vi "sub_associate_token.vi"(8 "error in":errorcluster, 9 "save to device?":bool=TRUE, 10 "device_id":string, 11 "daq.io type in":T1) -> (0 "error out":errorcluster, 3 "daq.io type out":T1={"daq.io ref"=refnum, "daq.io API Base"="http://dashboard.daq.io/api/v1", "Device Key"="", "Account ID"="", "online"=TRUE, "SSL"=TRUE})   [LabVIEW 2013, in "daqio minimal.lvlib"]
doc: "This VI associates the current token with the specified device. If \"save to device\" is true, it will also register the token on the device (default behavior)"
uses:
  daqio minimal.lvlib
  _typedefs/daqio-Type.ctl
  <vilib>/httpClient/ClientHandle.ctl
  <vilib>/Easy HTTP Client/Easy HTTP.lvlib
  <vilib>/httpClient/LabVIEWHTTPClient.lvlib
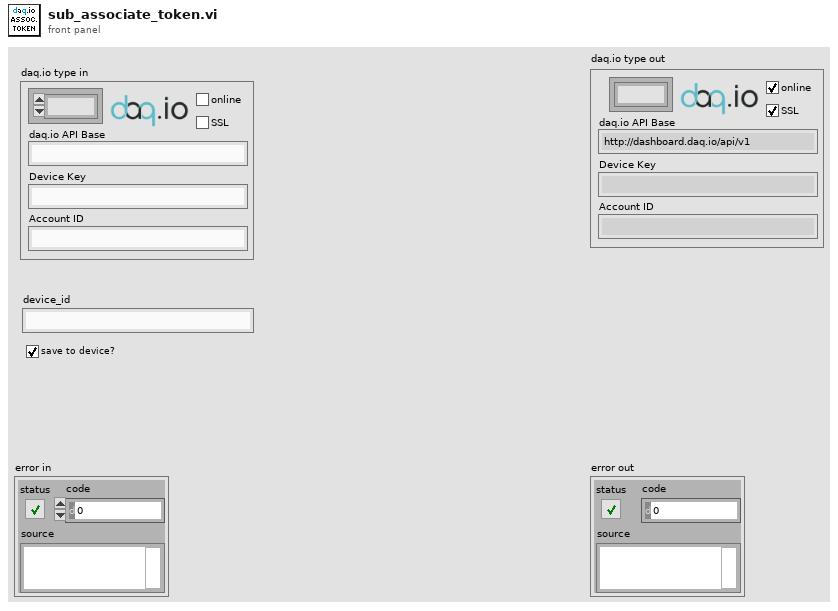
[diagram p1: front panel]
types:
  T1 = typedef "daqio minimal.lvlib/daqio-Type.ctl" = cluster{"daq.io ref":T2, "daq.io API Base":string, "Device Key":string, "Account ID":string, "online":bool, "SSL":bool}
  T2 = typedef "LabVIEWHTTPClient.lvlib/ClientHandle.ctl" = refnum<k1>
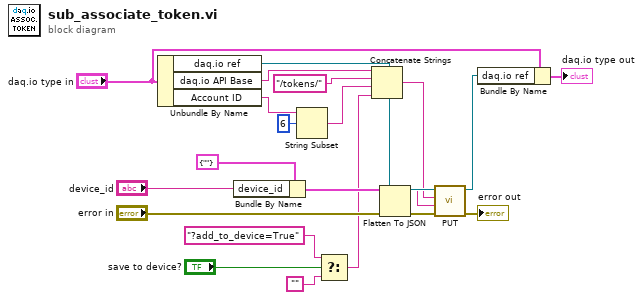
[diagram p0: block diagram]
diagram:
  n1 = Unbundle By Name("daq.io type in") -> ("daq.io ref"=w21:T2, "daq.io API Base"=w8:string, "Account ID"=w9:string)
  n2 = Bundle By Name(cluster=cluster{"device_id":string} {"device_id"=""}, "device_id"="device_id") -> (w17:cluster{"device_id":string})
  n3 = String Subset(string=w9, offset (0)=6) -> (substring=w12:string)  [unwired: 1 in]
  n4 = Select(t="?add_to_device=True" ("string"), s="save to device?", f="") -> (s? t:f=w1:string)
  n5 = Concatenate Strings(w8, "/tokens/" ("string"), w12, w1) -> (w13:string)
  n6 = Flatten To JSON(anything=w17, error in (no error)="error in") -> (JSON string=w18:string, 11:w19:errorcluster)  [unwired: 1 in]
  n7 = call <vilib>:"PUT.vi"("error in (no error)"=w19, "data"=w18, "url"=w13, "client handle"=w21) -> ("error out"=→"error out":errorcluster, "client handle out"=w6:T2)  [unwired: 3 in, 3 out]
  n8 = Bundle By Name(cluster="daq.io type in", "daq.io ref"=w6) -> (→"daq.io type out":T1)
